vi "LAB1_pt2_ex1.vi"() -> ()   [LabVIEW 2015]
doc: "This example demonstrates how to read N channels of analog input from a LINX device."
uses:
  <vilib>/MakerHub/LINX/Public/Peripherals/PWM/PWM Set Duty Cycle 1 Chan.vi
  <vilib>/MakerHub/LINX/Public/Peripherals/Digital/Digital Write 1 Chan.vi
  <vilib>/MakerHub/LINX/Public/Peripherals/Digital/Digital Write N Chans.vi
  <vilib>/MakerHub/LINX/Private/Local IO/LinxDigitalWrite.vi
  <vilib>/MakerHub/LINX/Public/Utilities/Check Channel.vi
  <vilib>/MakerHub/LINX/Public/Utilities/Open Serial.vi
  <vilib>/MakerHub/LINX/Public/Peripherals/PWM/PWM Set Duty Cycle N Chans.vi
  <vilib>/MakerHub/LINX/Private/Utilties/Generate Error.vi
  <vilib>/MakerHub/LINX/LMH-LINX.lvlib
panel:
  in  "?":dbl
  in  "Stop Button":bool
  in  "Serial Port":refnum<visa-resource-name>
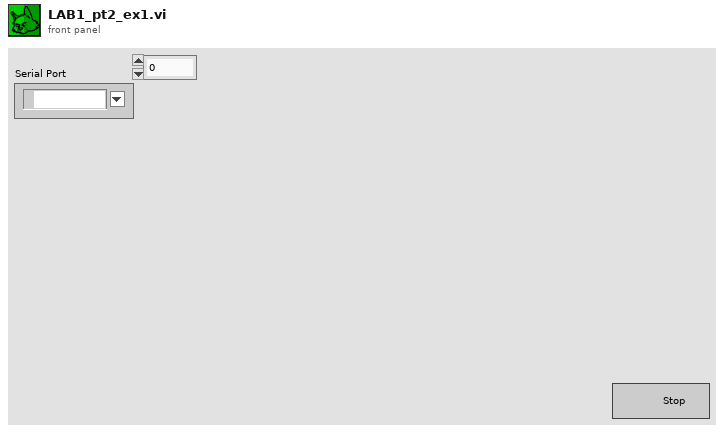
[diagram p1: front panel]
types:
  T1 = typedef "LMH-LINX.lvlib/LINX Ref.ctl" = cluster{"IO":T2, "Interface":T3, "LINX Device Config":T4}
  T2 = typedef "LMH-LINX.lvlib/Platform.ctl" = enum16{"Remote", "Local"}
  T3 = typedef "LMH-LINX.lvlib/Interface.ctl" = enum16{"Serial", "TCP"}
  T4 = typedef "LMH-LINX.lvlib/Device.lvlib/LINX Device Config.ctl" = cluster{"Interface":T3, "COM Port":refnum<visa-resource-name>, "TCP Configuration":T5, "Device Family":u8, "Device ID":u8, "Device Name":string, "TCP Ref":refnum<k5>, "Channels":T6}
  T5 = typedef "LMH-LINX.lvlib/Device.lvlib/TCP Config.ctl" = cluster{"IP Address":string, "Port":u16}
  T6 = typedef "LMH-LINX.lvlib/Channels.ctl" = cluster{"DI":u8[], "DO":u8[], "AI":u8[], "AO":u8[], "PWM":u8[], "QE":u8[], "UART":u8[], "I2C 2":u8[], "SPI":u8[], "CAN":u8[], "Servo":u8[], "AI Ref (V)":dbl, "AI Resolution (Bits)":u8, "AO Ref (V)":dbl, "AO Resolution (Bits)":u8}
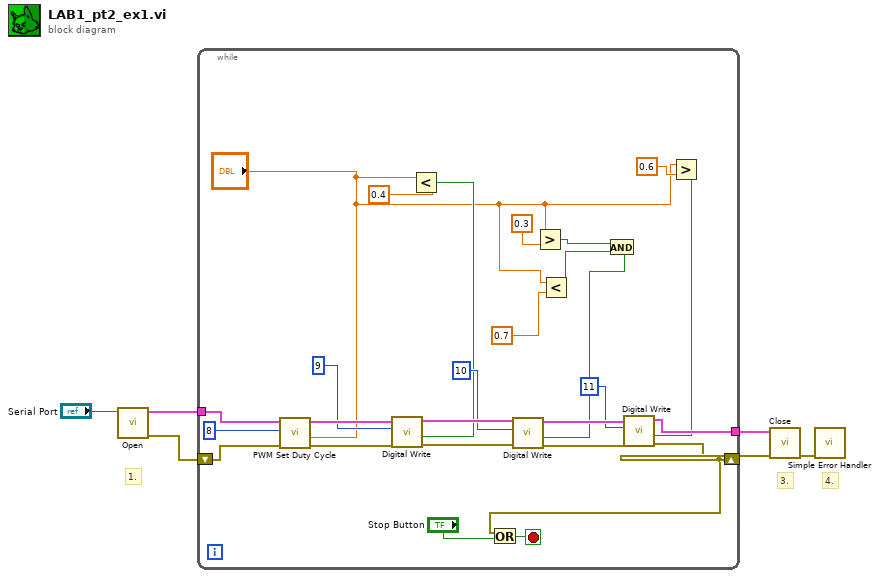
[diagram p0: block diagram]
diagram:
  # "4."
  # "3."
  # "1."
  n1 = call-poly <vilib>:"Open.vi"("Serial Port"="Serial Port") -> ("Error Out"=w5:errorcluster, "LINX Resource"=w6:T1)  [unwired: 8 in, 1 out]
  n2 = while {
    tunnel: w6 -> [w29]
    shift-right: [w20] -> w4
    shift-left: w5 -> [w28]
    tunnel: [w24] -> w1
    stop <- w32 stop-if-true
    n3 = call-poly <vilib>:"PWM Set Duty Cycle.vi"("Error In"=w28, "Duty Cycle (0-1)"="?", "PWM Channel"=8, "LINX Resource"=w29) -> ("Error Out"=w23:errorcluster, "LINX Resource"=w27:T1)  [unwired: 6 in]
    n4 = Less?(x="?", y=0.4) -> (x < y?=w11:bool)
    n5 = call-poly <vilib>:"Digital Write.vi"("Error In"=w23, "Output Value"=w11, "DO Channel"=9, "LINX Resource"=w27) -> ("Error Out"=w22:errorcluster, "LINX Resource"=w26:T1)  [unwired: 6 in]
    n6 = Greater?(x="?", y=0.3) -> (0:w12:bool)
    n7 = Less?(x="?", y=0.7) -> (x < y?=w10:bool)
    n8 = And(x=w12, y=w10) -> (x .and. y?=w9:bool)
    n9 = call-poly <vilib>:"Digital Write.vi"("Error In"=w22, "Output Value"=w9, "DO Channel"=10, "LINX Resource"=w26) -> ("Error Out"=w21:errorcluster, "LINX Resource"=w25:T1)  [unwired: 6 in]
    n10 = Greater?(x="?", y=0.6) -> (0:w16:bool)
    n11 = call-poly <vilib>:"Digital Write.vi"("Error In"=w21, "Output Value"=w16, "DO Channel"=11, "LINX Resource"=w25) -> ("Error Out"=w20:errorcluster, "LINX Resource"=w24:T1)  [unwired: 6 in]
    n12 = Or(x=w20, y="Stop Button") -> (x .or. y?=w32:bool)
  }
  n13 = call <vilib>:"Close.vi"("Error In"=w4, "LINX Resource"=w1) -> ("Error Out"=w2:errorcluster)  [unwired: 9 in]
  n14 = call <vilib>:"Simple Error Handler.vi"("error in (no error)"=w2) -> ()  [unwired: 4 in, 5 out]
